vi "Parse Cluster Z.vi"(3 "error in":T1, 4 "floating-point type conversion":string[][](table)=[["extended", "5", "12"], ["double", "5", "9"], ["single", "5", "5"]], 5 "cluster data":string, 6 "cluster definition":u16[](array[numeric])) -> (0 "error out":T1, 1 "cluster controls":T2(array[cluster]), 2 "cluster name":string)   [LabVIEW 2016]
doc: "Determines a cluster name, control names, controls types and control data values from a flattened cluster.\nModified from the original SQL add-on version, to save floating-point numbers in exponential format. The Parse Control Data subVI is replaced with an altered version."
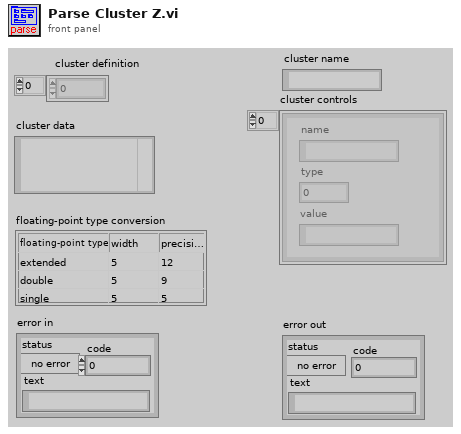
[diagram p1: front panel]
types:
  T1 = cluster{"status":bool, "code":i32, "text":string}
  T2 = cluster{"name":string, "type  ":u16, "value":string}[]
  T3 = cluster{"control name":string, "control type":u16, "data value":string}[]
  T4 = cluster{"control name":string, "control type":u16, "data value":string}
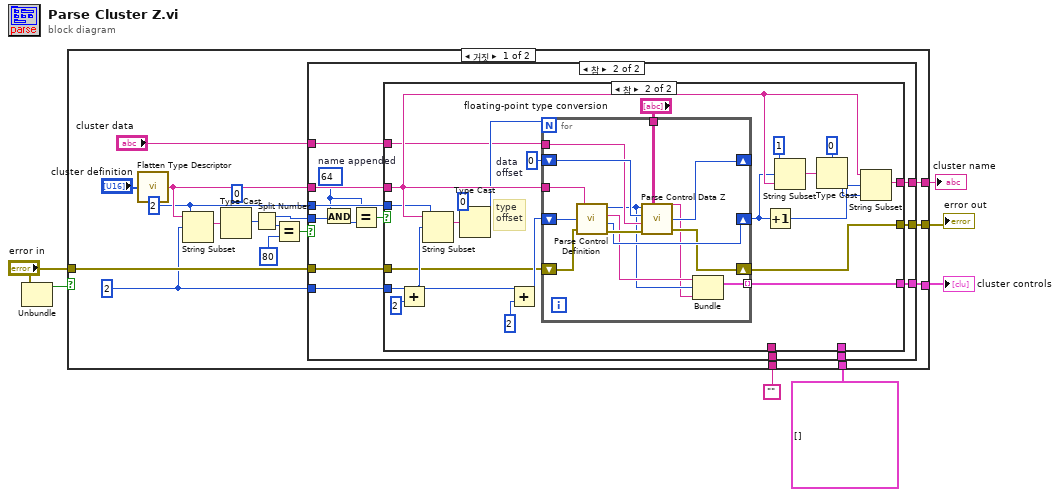
[diagram p0: block diagram]
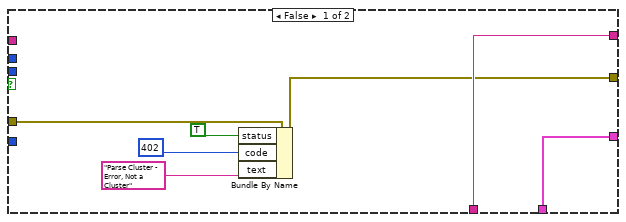
[diagram p2: hidden frame]
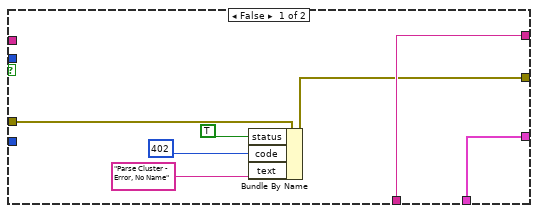
[diagram p3: hidden frame]
diagram:
  n1 = Unbundle("error in") -> ("status"=w6:bool)  [unwired: 2 out]
  n2 = case shown="거짓" w6 {
    tunnel: "error in" -> [w16 w93]
    tunnel: [w24 w93] -> w3
    tunnel: [w23 w91] -> w5
    tunnel: [w22 w92] -> w4
    tunnel: T3 [] -> [w18 w92]
    tunnel: "" -> [w17 w91]
    frame False {
      w19 = 2 ("offset (0)")
      w9 = 2 ("offset (0)")
      n3 = call <vilib>:"Flatten Type Descriptor.vi"("type descriptor"="cluster definition") -> ("flattened type descriptor"=w20:string)  [unwired: 4 in]
      n4 = String Subset(string=w20, offset (0)=w9, length (rest)=w19) -> (substring=w14:string)
      n5 = Type Cast(type=u16 0 ("offset (0)"), x=w14) -> (*(type *) &x=w11:u16)
      n6 = Split Number(x=w11) -> (hi(x)=w8:u8, lo(x)=w10:u8)
      n7 = Equal?(x=w10, y=u16 80 ("offset (0)")) -> (x = y?=w13:bool)
      n8 = case shown="참" w13 {
        tunnel: w19 -> [_ w46]
        tunnel: w20 -> [_ w40]
        tunnel: [w32 w45] -> w22
        tunnel: [w31 w41] -> w23
        tunnel: [w29 w42] -> w24
        tunnel: "cluster data" -> [_ w44]
        tunnel: w18 -> [w32 w33]
        tunnel: w17 -> [w31 w34]
        tunnel: w16 -> [w30 w43]
        tunnel: w9 -> [_ w39]
        tunnel: w8 -> [_ w38]
        frame False {
          n9 = Bundle By Name(cluster=w30, "status"=TRUE, "code"=402, "text"="Parse Cluster - Error, Not a Cluster") -> (w29:T1)
        }
        frame True {
          w36 = u8 64  # name appended
          n10 = And(x=w36, y=w38) -> (x .and. y?=w37:u8)
          n11 = Equal?(x=w36, y=w37) -> (x = y?=w35:bool)
          n12 = case shown="참" w35 {
            tunnel: w39 -> [_ w72]
            tunnel: w40 -> [_ w70]
            tunnel: [w53 w64] -> w41
            tunnel: [w47 w63] -> w42
            tunnel: w43 -> [w48 w59]
            tunnel: w44 -> [_ w57]
            tunnel: [w52 w55] -> w45
            tunnel: w46 -> [_ w54]
            tunnel: w34 -> [w53 _]
            tunnel: w33 -> [w52 _]
            frame False {
              n13 = Bundle By Name(cluster=w48, "status"=TRUE, "code"=402, "text"="Parse Cluster - Error, No Name") -> (w47:T1)
            }
            frame True {
              w58 = 0  # data offset
              # "type\noffset"
              n14 = Add(x=w72, y=2 ("offset (0)")) -> (x+y=w75:i32)
              n15 = String Subset(string=w70, offset (0)=w75, length (rest)=w54) -> (substring=w60:string)
              n16 = Type Cast(type=u16 0 ("offset (0)"), x=w60) -> (*(type *) &x=w62:u16)
              n17 = Add(x=w75, y=2 ("offset (0)")) -> (x+y=w76:i32)
              n18 = for {
                N: w62 -> [_]
                shift-right: [w83] -> w68
                shift-left: w76 -> [w90]
                shift-right: [w84] -> _
                shift-left: w58 -> [w88]
                shift-right: [w82] -> w63
                shift-left: w59 -> [w89]
                tunnel: w57 -> [w87]
                tunnel: "floating-point type conversion" -> [w86]
                tunnel: [w81] -> w55 mode=indexing
                tunnel: w70 -> [w77]
                n19 = call <vilib>:"Parse Control Definition.vi"("cluster type descriptor"=w77, "offset"=w90, "error in"=w89) -> ("control type"=w79:u16, "control name"=w80:string, "offset past control"=w83:i32, "error out"=w85:errorcluster)
                n20 = call "Parse Control Data Z.vi"("control type"=w79, "offset"=w88, "cluster data"=w87, "error in"=w85, "floating-point type conversion"=w86) -> ("data value"=w78:string, "offset past cluster data"=w84:i32, "error out"=w82:T1)
                n21 = Bundle("control name"=w80, "control type"=w79, "data value"=w78) -> (w81:T4)  [unwired: 1 in]
              }
              n22 = Increment(x=w68) -> (x+1=w71:i32)
              n23 = String Subset(string=w70, offset (0)=w68, length (rest)=1 ("offset (0)")) -> (substring=w67:string)
              n24 = Type Cast(type=u8 0 ("offset (0)"), x=w67) -> (*(type *) &x=w69:u8)
              n25 = String Subset(string=w70, offset (0)=w71, length (rest)=w69) -> (substring=w64:string)
            }
          }
        }
      }
    }
    frame True {
    }
  }
  "cluster name" <- w5
  "error out" <- w3
  "cluster controls" <- w4
